vi "Ignore Fail.vi"(8 "error in (no error)":errorcluster, 10 "IgnoreFail":bool, 11 "Algorithm in":refnum<class "Algorithm.lvclass">) -> (0 "error out":errorcluster, 3 "Algorithm out":refnum<class "Algorithm.lvclass">)   [LabVIEW 2015, in "Algorithm.lvclass"]
uses:
  FrameworkOverrides/Algorithm.lvclass
  <vilib>/event_ctls.llb/usereventprio.ctl
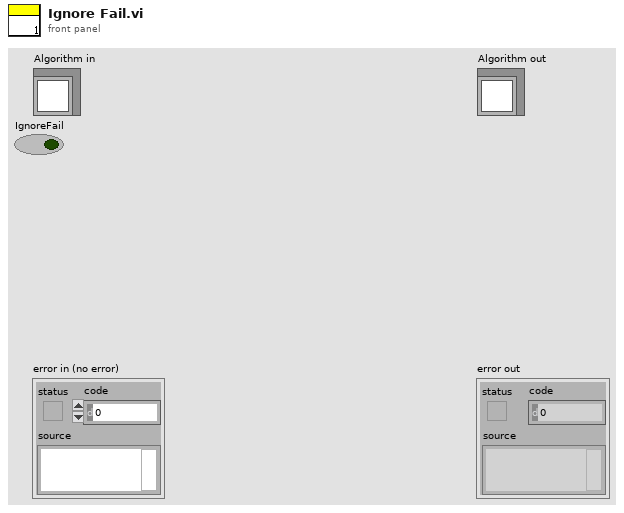
[diagram p1: front panel]
types:
  T1 = typedef "usereventprio.ctl" = enum32{"high priority", "normal priority"}
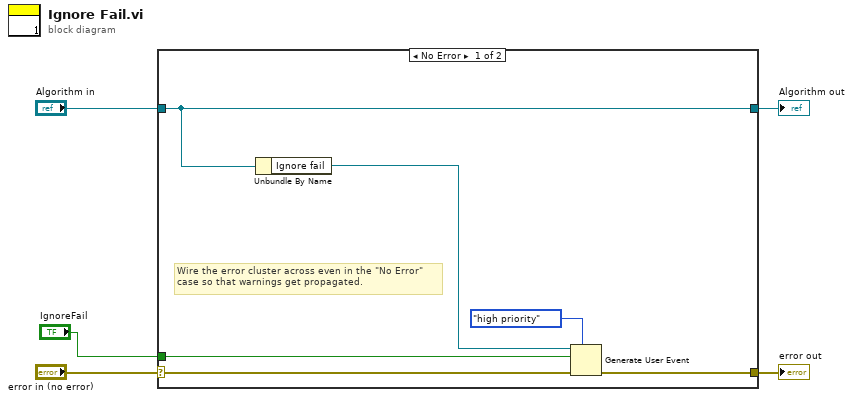
[diagram p0: block diagram]
diagram:
  n1 = case shown="No Error" "error in (no error)" {
    selector: "error in (no error)" -> [w10 w13]
    tunnel: [w9 w13] -> w4
    tunnel: [w11 w12] -> w2
    tunnel: "Algorithm in" -> [w11 w12]
    tunnel: "IgnoreFail" -> [w6 _]
    frame No Error {
      # "Wire the error cluster across even in the \"No Error\"\ncase so that warnings get propagated."
      n2 = Unbundle By Name(w11) -> ("Ignore fail"=w8:refnum<user-event>)
      n3 = Generate User Event(priority (normal)=usereventprio."high priority", user event=w8, event data cluster=w6, error in=w10) -> (error out=w9:errorcluster)  [unwired: 1 out]
    }
    frame Error {
    }
  }
  "error out" <- w4
  "Algorithm out" <- w2
